vi "Kinesis - KDC101 - Motor Status Changed (Callback VI).vi"(4 "User Parameter":variant, 5 "Event Data":cluster{"sender":refnum<k24>, "e":refnum<k24>}, 6 "Control Ref":refnum<k24>, 7 "Event Common Data":T1) -> ()   [LabVIEW 2019]
uses:
  C:/Program Files (x86)/National Instruments/LabVIEW 2019/user.lib/ThorKDC101/Kinesis_with_LabVIEW_Examples_LV12 - v3/Thorlabs.MotionControl.GenericMotorCLI.dll
  Thorlabs.MotionControl.GenericMotorCLI.dll
panel:
  # "Please refer to the \"Kinesis - KDC101 - Motor Status Changed.vi\" for instructions."
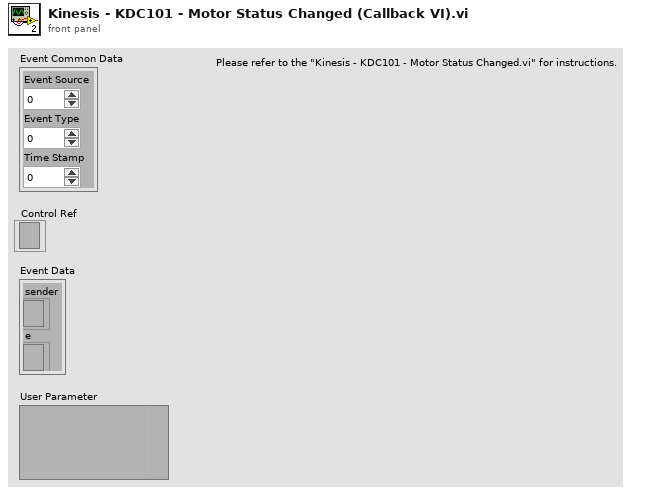
[diagram p1: front panel]
types:
  T1 = cluster{"Event Source":i32, "Event Type":u32, "Time Stamp":u32}
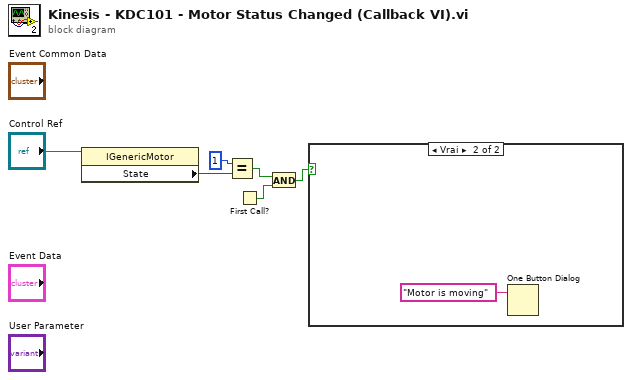
[diagram p0: block diagram]
diagram:
  n1 = property class="IGenericMotor"(reference="Control Ref") -> ("State"=w5:i32)  [unwired: 1 in, 2 out]
  n2 = Equal?(x=1, y=w5) -> (x = y?=w2:bool)
  n3 = First Call?() -> (First Call?: T/F=w3:bool)
  n4 = And(x=w2, y=w3) -> (x .and. y?=w1:bool)
  n5 = case shown="Vrai" w1 {
    frame False {
    }
    frame True {
      n6 = One Button Dialog(message="Motor is moving") -> ()  [unwired: 1 in, 1 out]
    }
  }
